vi "VCM_Split_Cluster.vi"(0 "VCM Monitor":T3) -> (1 "VCM Status":T1, 2 "VCM Control":T2)   [LabVIEW 2019]
uses:
  Mischer/VCM-Cluster.ctl
  Mischer/VCM-Control.ctl
  Mischer/VCM-Status.ctl
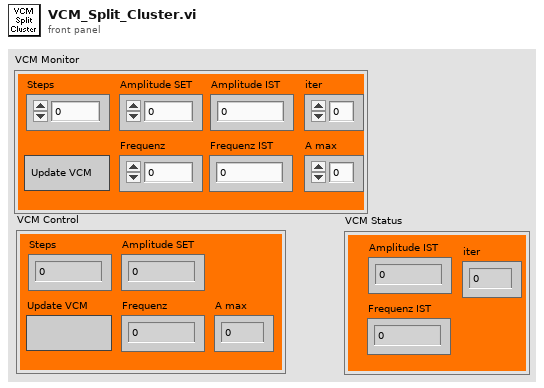
[diagram p1: front panel]
types:
  T1 = typedef "VCM-Status.ctl" = cluster{"Amplitude IST":dbl, "Frequenz IST":dbl, "iter":dbl}
  T2 = typedef "VCM-Control.ctl" = cluster{"Steps":dbl, "Amplitude SET":dbl, "Frequenz":dbl, "A max":dbl, "Update VCM":bool}
  T3 = typedef "VCM-Cluster.ctl" = cluster{"Steps":dbl, "Amplitude SET":dbl, "Frequenz":dbl, "Amplitude IST":dbl, "Frequenz IST":dbl, "A max":dbl, "iter":dbl, "Update VCM":bool}
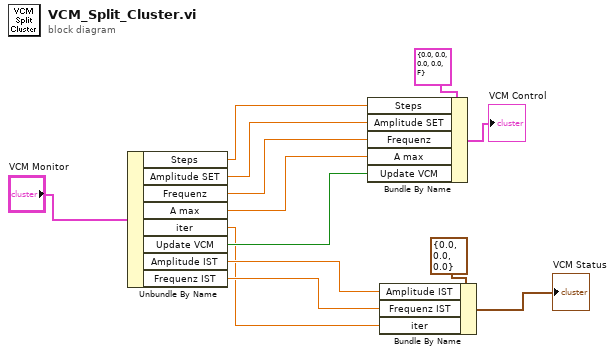
[diagram p0: block diagram]
diagram:
  n1 = Unbundle By Name("VCM Monitor") -> ("Steps"=w8:dbl, "Amplitude SET"=w7:dbl, "Frequenz"=w6:dbl, "A max"=w5:dbl, "iter"=w1:dbl, "Update VCM"=w4:bool, "Amplitude IST"=w3:dbl, "Frequenz IST"=w2:dbl)
  n2 = Bundle By Name(cluster=T2 {"Steps"=0.0, "Amplitude SET"=0.0, "Frequenz"=0.0, "A max"=0.0, "Update VCM"=FALSE} ("VCM Control"), "Steps"=w8, "Amplitude SET"=w7, "Frequenz"=w6, "A max"=w5, "Update VCM"=w4) -> (→"VCM Control":T2)
  n3 = Bundle By Name(cluster=T1 {"Amplitude IST"=0.0, "Frequenz IST"=0.0, "iter"=0.0} ("VCM Staus"), "Amplitude IST"=w3, "Frequenz IST"=w2, "iter"=w1) -> (→"VCM Status":T1)
